vi "Test Program  Updated.vi"() -> ()   [LabVIEW 2018, in "VICI M6 M50 Party Mode.lvlib"]
uses:
  VICI M6 M50 Party Mode.lvlib
  Settings Cluster.ctl
panel:
  out "read buffer 2":string
  out "Pump On?":enum16{"Off", "On", "Not Initialized"}(ring)
  in  "stop":bool
  in  "speed":dbl
  in  "VICI Settings":T1
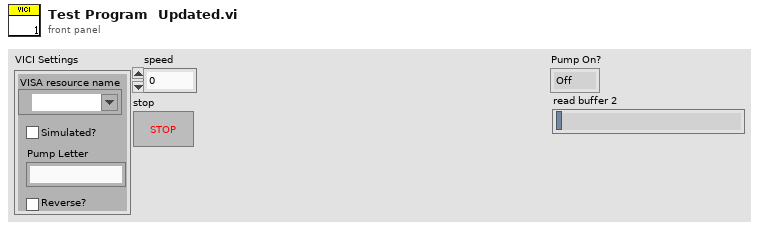
[diagram p1: front panel]
types:
  T1 = typedef "VICI M6 M50 Party Mode.lvlib/Settings Cluster.ctl" = cluster{"VISA resource name":refnum<visa-resource-name>, "Simulated?":bool, "Pump Letter":string, "Reverse?":bool}
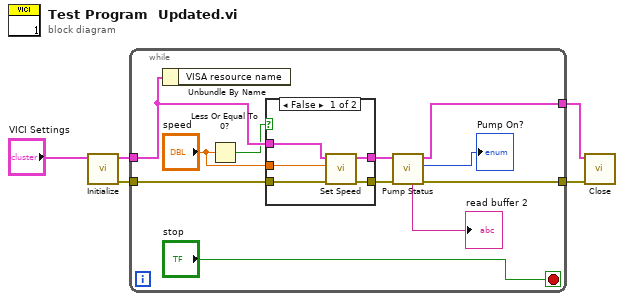
[diagram p0: block diagram]
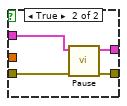
[diagram p2: hidden frame]
diagram:
  n1 = call "Initialize.vi"("VICI Settings"="VICI Settings") -> ("error out"=w2:errorcluster, "VICI Settings"=w4:T1)  [unwired: 7 in, 2 out]
  n2 = while {
    tunnel: w4 -> [w11]
    tunnel: [w15] -> w3
    tunnel: w2 -> [w14]
    tunnel: [w12] -> w1
    stop <- "stop" stop-if-true
    n3 = Unbundle By Name(w11) -> ()  [unwired: 1 out]
    n4 = Less Or Equal To 0?(x="speed") -> (x <= 0?=w9:bool)
    n5 = case shown="False" w9 {
      tunnel: w11 -> [w21 w25]
      tunnel: [w20 w24] -> w16
      tunnel: w14 -> [w18 w23]
      tunnel: [w19 w22] -> w13
      tunnel: "speed" -> [w17 _]
      frame False {
        n6 = call "Set Speed.vi"("error in (no error)"=w18, "speed"=w17, "VICI Settings"=w21) -> ("error out"=w19:errorcluster, "VICI Settings"=w20:T1)  [unwired: 6 in, 1 out]
      }
      frame True {
        n7 = call "Pause.vi"("error in (no error)"=w23, "VICI Settings"=w25) -> ("error out"=w22:errorcluster, "VICI Settings"=w24:T1)  [unwired: 7 in, 1 out]
      }
    }
    n8 = call "Pump Status.vi"("error in (no error)"=w13, "VICI Settings"=w16) -> ("error out"=w12:errorcluster, "Pump On?"=→"Pump On?":enum16{"Off", "On", "Not Initialized"}, "VICI Settings"=w15:T1, "read buffer 2"=→"read buffer 2":string)  [unwired: 5 in, 1 out]
  }
  n9 = call "Close.vi"("error in (no error)"=w1, "VICI Settings"=w3) -> ()  [unwired: 7 in, 3 out]
